vi "SetParam.vi"(8 "error in (no error)":errorcluster caption="entrée d'erreur (pas d'erreur)", 10 "PredefinedSplit":cluster{"test_fold":dbl[]}, 11 "PredefinedSplit.lvclass":refnum<class "PredefinedSplit.lvclass">) -> (0 "error out":errorcluster caption="sortie d'erreur", 3 "PredefinedSplit.lvclass":refnum<class "PredefinedSplit.lvclass">)   [LabVIEW 2020, in "PredefinedSplit.lvclass"]
doc: "Set Parameters"
uses:
  PredefinedSplit.lvclass
  PredefinedSplit.lvclass/PredefinedSplit.ctl
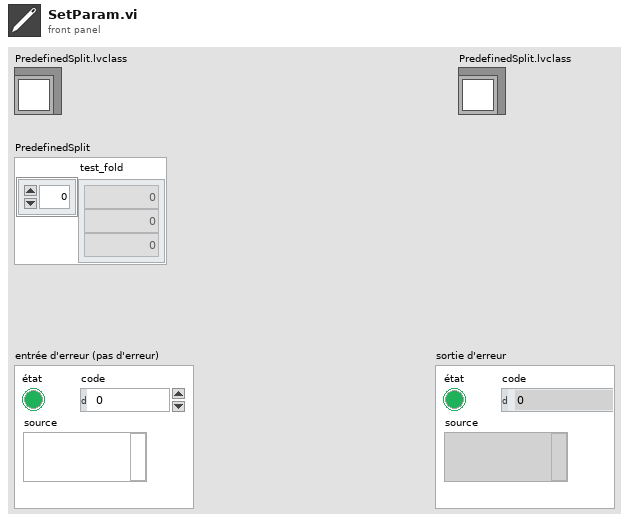
[diagram p1: front panel]
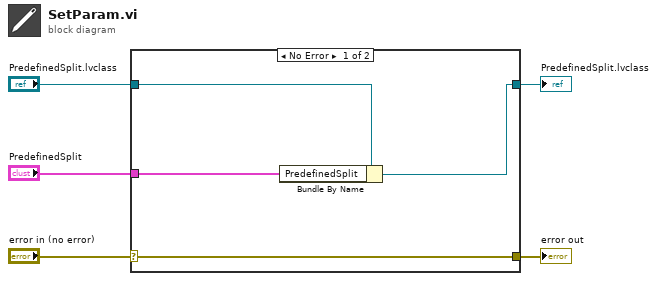
[diagram p0: block diagram]
diagram:
  n1 = case shown="No Error" "error in (no error)" {
    selector: "error in (no error)" -> [w9 w10]
    tunnel: [w9 w10] -> w4
    tunnel: [w7 w11] -> w2
    tunnel: "PredefinedSplit.lvclass" -> [w8 w11]
    tunnel: "PredefinedSplit" -> [w6 _]
    frame No Error {
      n2 = Bundle By Name(cluster=w8, "PredefinedSplit"=w6) -> (w7:refnum<class "PredefinedSplit.lvclass">)
    }
    frame Error {
    }
  }
  "error out" <- w4
  "PredefinedSplit.lvclass" <- w2
